vi "reference construction_forpicread(subVI).vi"(11 "Image in":T1) -> (0 "Waveform Graph 2":dbl[](graph), 1 "error out":errorcluster, 2 "Amplitudes":dbl[](array[numeric]) format="%.2p", 3 "Locations":dbl[](array[numeric]) format="%.2p", 4 "Power Spectrum":dbl[](array[numeric]))   [LabVIEW 2014]
doc: "This VI analyzes input stuck bead image with the following processes: \n1. Detect the multiple ring center and radius of stuck bead pattern. \n2. Read the intensity of the line across the stuck bead ring pattern image. \n3. Calculate the FT of intensity of ring pattern by power spectrum. \n4. Find peak on the FT plot and output peak locations & amplitudes."
uses:
  <vilib>/vision/Image Controls.llb/IMAQ Image.ctl
panel:
  out "PSD":dbl[](graph)
  in  "BCG Values":T2={"Brightness"=200.0, "Contrast"=50.0, "Gamma"=2.9999995}
  in  "adjust constrast?":bool
  out "Extract Image":T1(plugin-control)
  out "# found":i32
  out "Waveform Graph":u8[](graph)
  out "Pixels Line (U8)":u8[](array[numeric])
  in  "Remaining Inputs":T3={"Circle Descriptor (Shape Detection 1)"={"Min Radius"=3.0, "Max Radius"=500.0}, "Y Scale.Mapping Mode (Line Profile 1)"=0}
  in  "Match Options (Shape Detection 1)":T4={"Rotation"=TRUE, "Scale"=FALSE, "Occlusion"=FALSE, "Range Settings"=[{"Match Constraints"=0, "Min"=0.0, "Max"=360.0}]} {"Range Settings"."Match Constraints" items=["Rotation Angle (degrees)", "Scale Factor (%)", "Occlusion (%)"]}
  in  "Minimum match score (Shape Detection 1)":dbl=800.0
  in  "Curve Parameters (Shape Detection 1)":T5={"Extraction Mode"=0, "Edge Threshold"=11, "Edge Filter Size"=1, "Min Length"=1, "Row Search Step Size"=1, "Col Search Step Size"=1, "Max Endpoint Gap"=1, "Closed"=FALSE, "Subpixel"=FALSE} {"Extraction Mode" items=["Normal", "Uniform Regions"]; "Edge Filter Size" items=["Fine", "Normal"]}
  in  "ROI Descriptor (Shape Detection 1)":T6={"Global Rectangle"=[6, 17, 113, 117], "Contours"=[{"ID"=enum."External", "Type"=3, "Coordinates"=[6, 17, 113, 117]}]} {"Contours"."Type" items=["No Selection", "Point", "Line", "Rectangle", "Oval", "Polygon", "Freehand Region", "Annulus", "Unused2", "Unused3", "Broken Line", "Freehand Line", "Rotated Rectangle"]}
  out "Circles (Shape Detection 1)":T7(array[cluster]) {"Position"."Y" format="%.2f"; "Position"."X" format="%.2f"}
  out "Number of Matches (Shape Detection 1)":i32
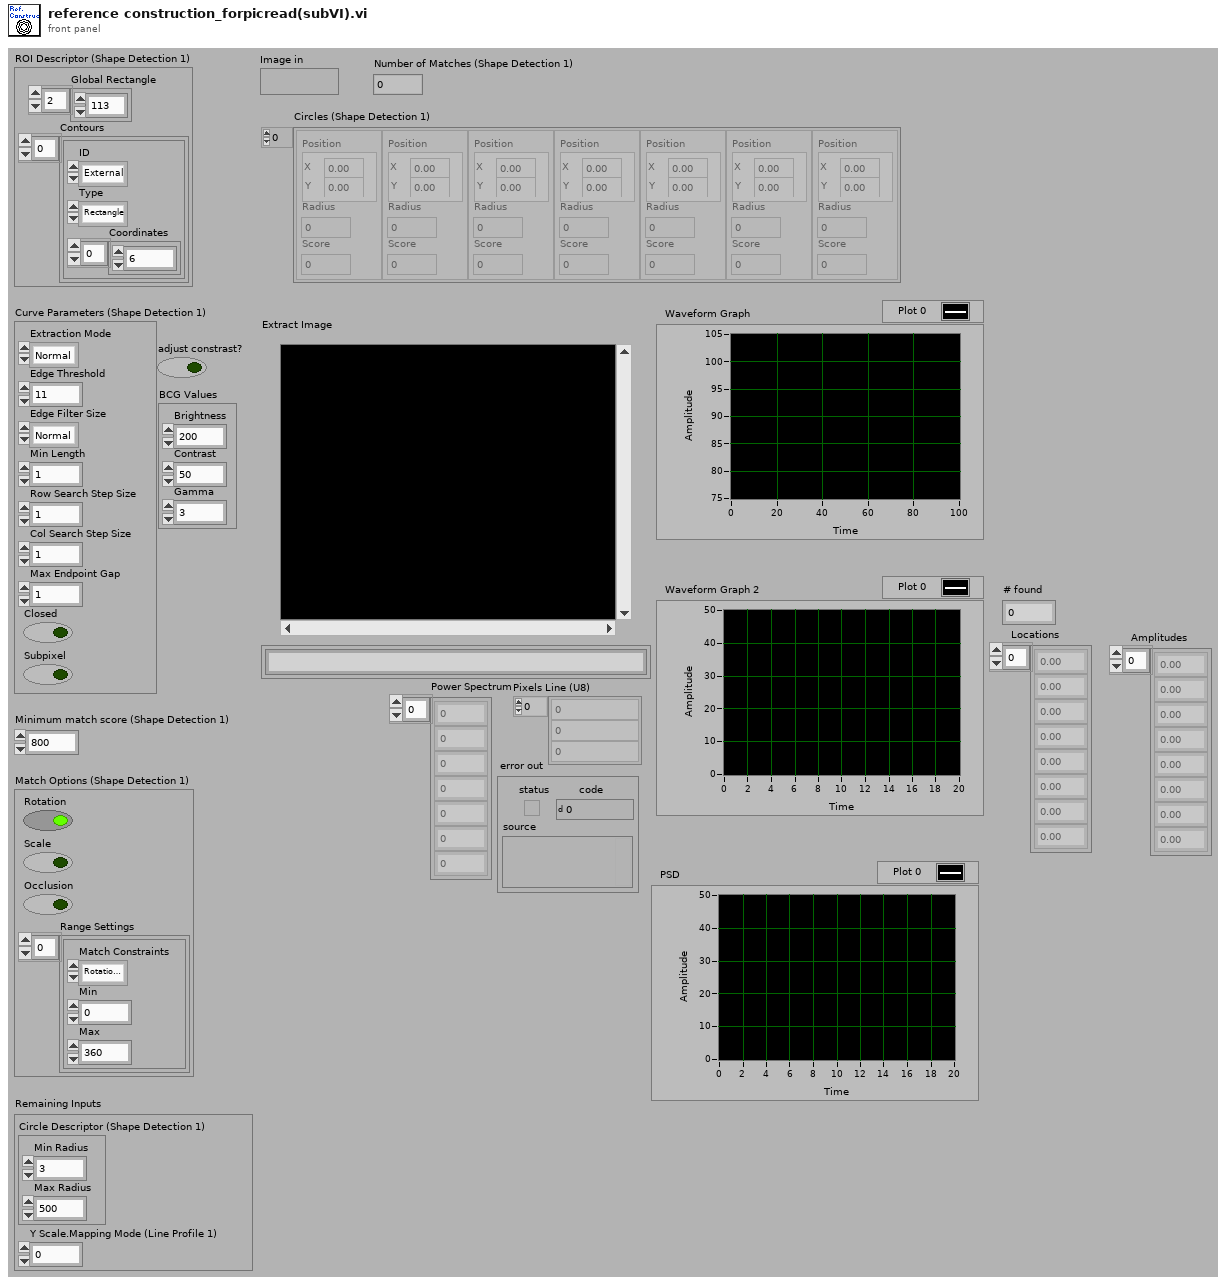
[diagram p1: front panel]
types:
  T1 = typedef "IMAQ Image.ctl" = refnum<image>
  T2 = cluster{"Brightness":sgl, "Contrast":sgl, "Gamma":sgl}
  T3 = cluster{"Circle Descriptor (Shape Detection 1)":cluster{"Min Radius":dbl, "Max Radius":dbl}, "Y Scale.Mapping Mode (Line Profile 1)":u8}
  T4 = cluster{"Rotation":bool, "Scale":bool, "Occlusion":bool, "Range Settings":cluster{"Match Constraints":u32, "Min":dbl, "Max":dbl}[]}
  T5 = cluster{"Extraction Mode":u32, "Edge Threshold":i32, "Edge Filter Size":u32, "Min Length":i32, "Row Search Step Size":i32, "Col Search Step Size":i32, "Max Endpoint Gap":i32, "Closed":bool, "Subpixel":bool}
  T6 = cluster{"Global Rectangle":i32[], "Contours":cluster{"ID":enum32{"External", "Internal"}, "Type":u32, "Coordinates":i32[]}[]}
  T7 = cluster{"Position":cluster{"X":sgl, "Y":sgl}, "Radius":dbl, "Score":dbl}[]
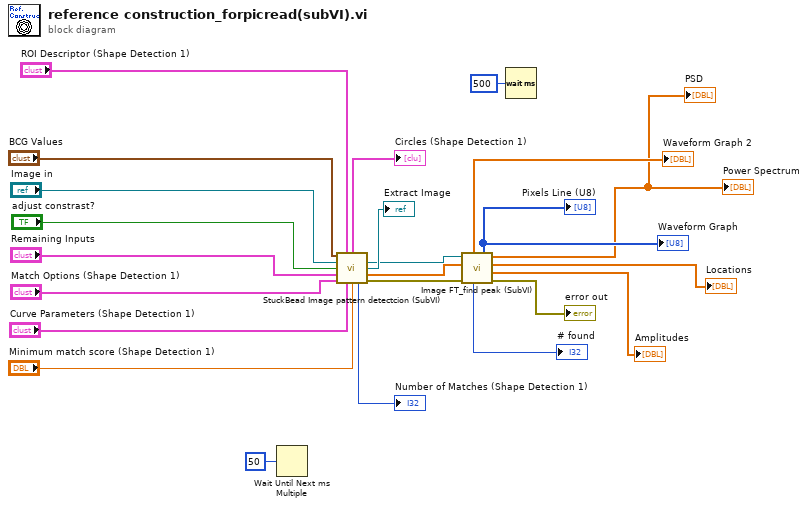
[diagram p0: block diagram]
diagram:
  n1 = Wait Until Next ms Multiple(millisecond multiple=u32 50) -> ()  [unwired: 1 out]
  n2 = call "StuckBead Image pattern detectcion (SubVI).vi"("BCG Values"="BCG Values", "ROI Descriptor (Shape Detection 1)"="ROI Descriptor (Shape Detection 1)", "Refnum in"="Image in", "adjust?"="adjust constrast?", "Remaining Inputs"="Remaining Inputs", "Match Options (Shape Detection 1)"="Match Options (Shape Detection 1)", "Curve Parameters (Shape Detection 1)"="Curve Parameters (Shape Detection 1)", "Minimum match score (Shape Detection 1)"="Minimum match score (Shape Detection 1)") -> ("Circles (Shape Detection 1)"=→"Circles (Shape Detection 1)":T7, "Refnum out"=w9:T1, "Image dup"=→"Extract Image":T1, "Array"=w10:sgl[], "Number of Matches (Shape Detection 1)"=→"Number of Matches (Shape Detection 1)":i32, "error out"=w12:errorcluster)  [unwired: 2 out]
  n3 = call "Image FT_find peak (SubVI).vi"("error in (no error)"=w12, "Array"=w10, "Refnum in"=w9) -> ("error out"=→"error out":errorcluster, "Amplitudes"=→"Amplitudes":dbl[], "Locations"=→"Locations":dbl[], "Power Spectrum"=→"Power Spectrum" →"PSD":dbl[], "Pixels Line (U8)"=→"Pixels Line (U8)" →"Waveform Graph":u8[], "# found"=→"# found":i32, "Waveform Graph 2"=→"Waveform Graph 2":dbl[])  [unwired: 2 in]
  n4 = Wait (ms)(milliseconds to wait=u32 500) -> ()  [unwired: 1 out]
